vi "ScanningWaveform_v6.vi"(0 "Vy-min":dbl, 1 "Vy-max":dbl, 2 "yPixels/tPixels":dbl, 3 "xPixels/rPixels":dbl, 4 "Vx-min":dbl, 5 "Vx-max":dbl, 6 "Drawing Mode":u16(ring) items=["Image", "Fill Rectangle", "Fill Circle", "Draw Freeform", "Fill Freeform", "Ellipse Boundary", "Line"], 7 "Angle":dbl, 8 "Scanning Mode":u16(ring) items=["Raster", "Spiral"], 9 "AOrate":dbl, 10 "Points":cluster{"X":dbl, "Y":dbl}[](array[cluster]), 11 "points in ellipse":dbl) -> (12 "numPixels":dbl, 13 "Y-WaveArray":dbl[](array[numeric]), 14 "P":dbl, 19 "X-WaveArray":dbl[](array[numeric]))   [LabVIEW 2015]
panel:
  out "Y Graph 4":dbl[][](graph)
  out "Y Graph 3":dbl[][](graph)
  out "X-Y Graph 3":T1(graph)
  out "Y Graph 2":dbl[](graph)
  out "X-Y Graph 2":cluster{dbl[], dbl[]}(graph)
  out "min":dbl
  out "max":dbl
  out "Points 2":cluster{"R":dbl, "Theta":dbl}[](array[cluster])
  out "X-Y Graph":cluster{dbl[], dbl[]}(graph)
  out "flyback time (us)":dbl
  out "Y Graph":dbl[](graph)
  out "X Graph":dbl[](graph)
  out "C":dbl
  out "Sx":dbl
  out "S":dbl
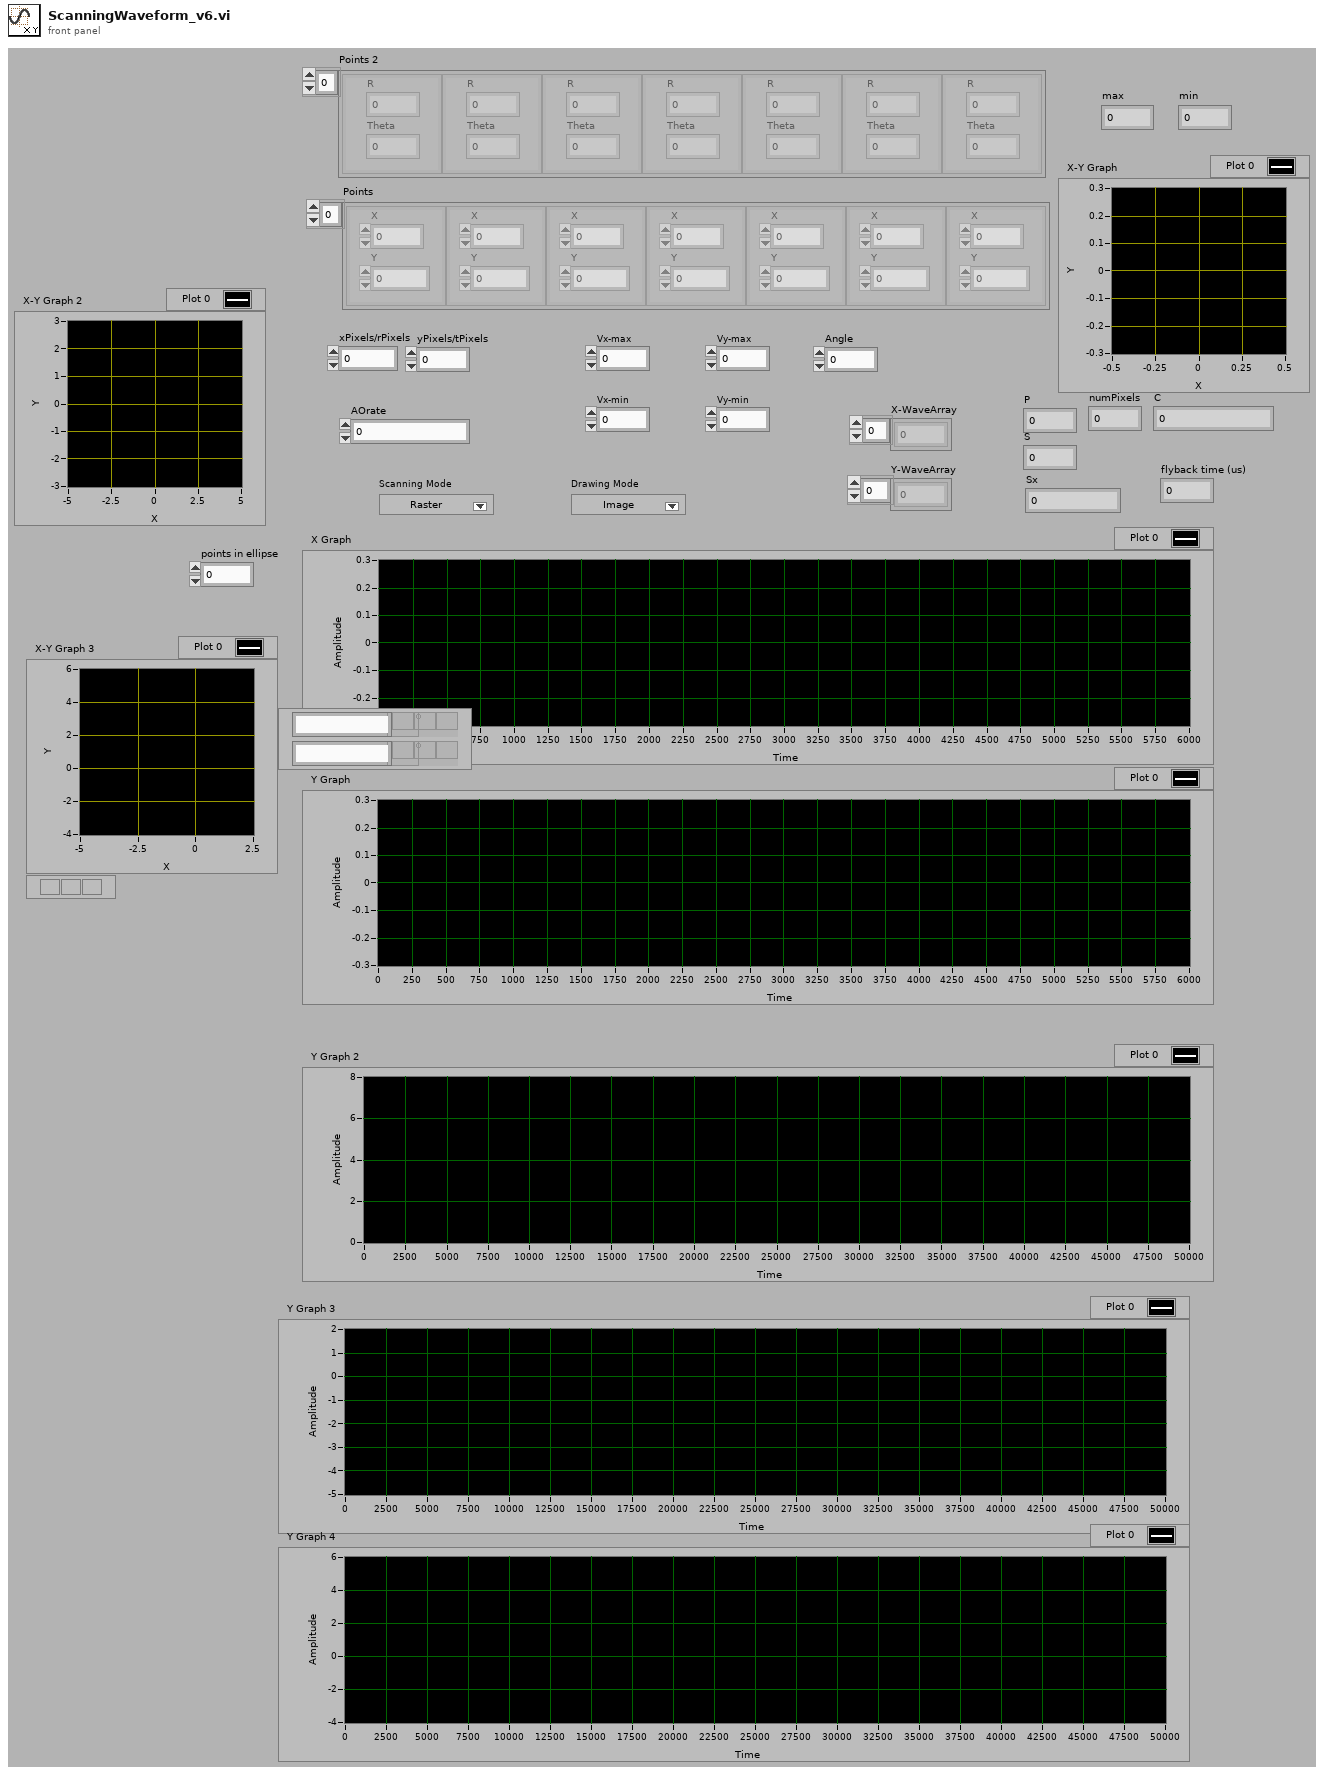
[diagram p1: front panel]
types:
  T1 = cluster{"X-WaveArray":dbl[], "Y-WaveArray":dbl[]}[]
  T2 = typedef "LVRectTypeDef.ctl" = cluster{"Left":i16, "Top":i16, "Right":i16, "Bottom":i16}
  T3 = cluster{"Xpixels":i32, "Vxminref":dbl, "Vxmaxref":dbl, "P":dbl, "Ypixels":i32, "Vyminref":dbl, "Vymaxref":dbl, "srate":sgl, "sAOxy":i32, "timeout":dbl, "type":string, "date":string, "time":string, "Colormap":u16, "Drawing Mode":u16, "Scanning Mode":u16, "square pixels":bool, "square matrix":bool, "Xpixels Img":i32, "Vx-min Img":dbl, "VX-max Img":dbl, "Ypixels Img":i32, "Vy-min Img":dbl, "Vy-max Img ":dbl, "Angle Img":dbl, "autoshutter":bool, "finite":bool, "cont":bool, "wavdet":bool, "measpoints":i32, "avpp":i32, "bufferAO":i32, "bufferAI":i32, "starttick":u32, "waveform":path, "Vx-ref":dbl, "Vy-ref":dbl, "refreshrate":dbl, "refreshbuffer":i32, "tt_cycles":i32, "motorref":refnum<k7>, "mirrorswitch":refnum<k7>, "sample mode":i32, "maxbufferAI":i32, "sampletreshold":dbl, "srateAODO":sgl, "bin":sgl, "Pel":sgl, "Angle draw":dbl, "srate Img":sgl, "ROIimg_plotbounds":T2, "auto OD":bool, "ODfilt":u16, "reset AO_DO":bool, "aAI":i32[], "aCI":i32[], "aAO":u32[], "aDO":u32[], "refwfsize":dbl, "Lifetime":bool, "Vz-Img":dbl, "Vz-ref":dbl, "Vz-reset":dbl}
  T4 = cluster{cluster{dbl, dbl}[], cluster{dbl, dbl}[]}
  T5 = cluster{"X-WaveArray":dbl[], "Y-WaveArray":dbl[]}
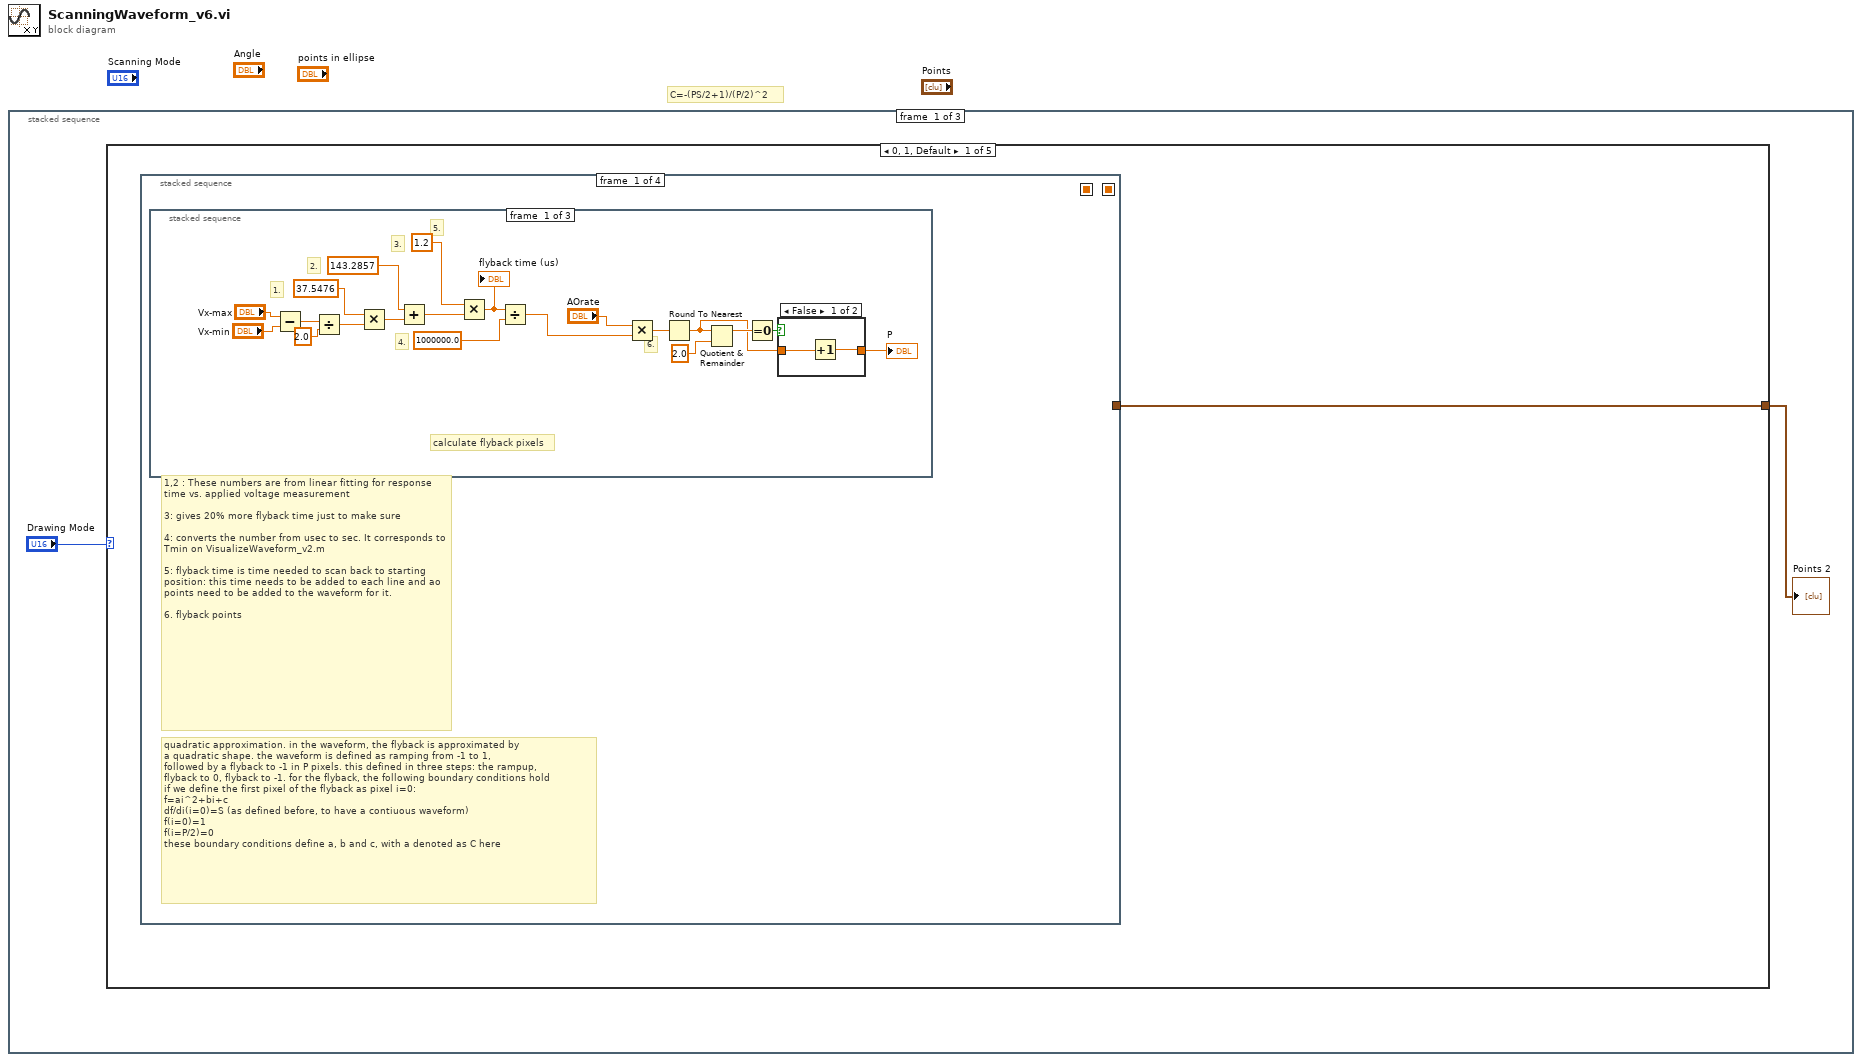
[diagram p0: block diagram]
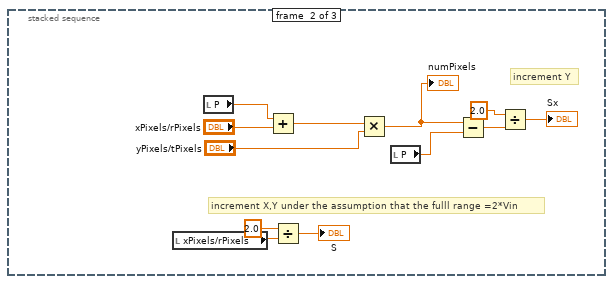
[diagram p3: hidden frame]
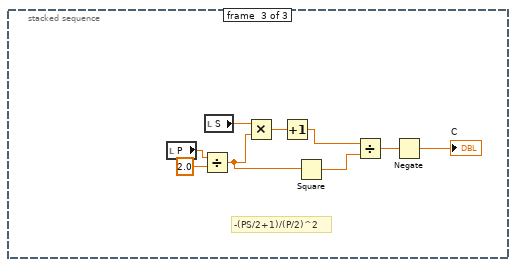
[diagram p4: hidden frame]
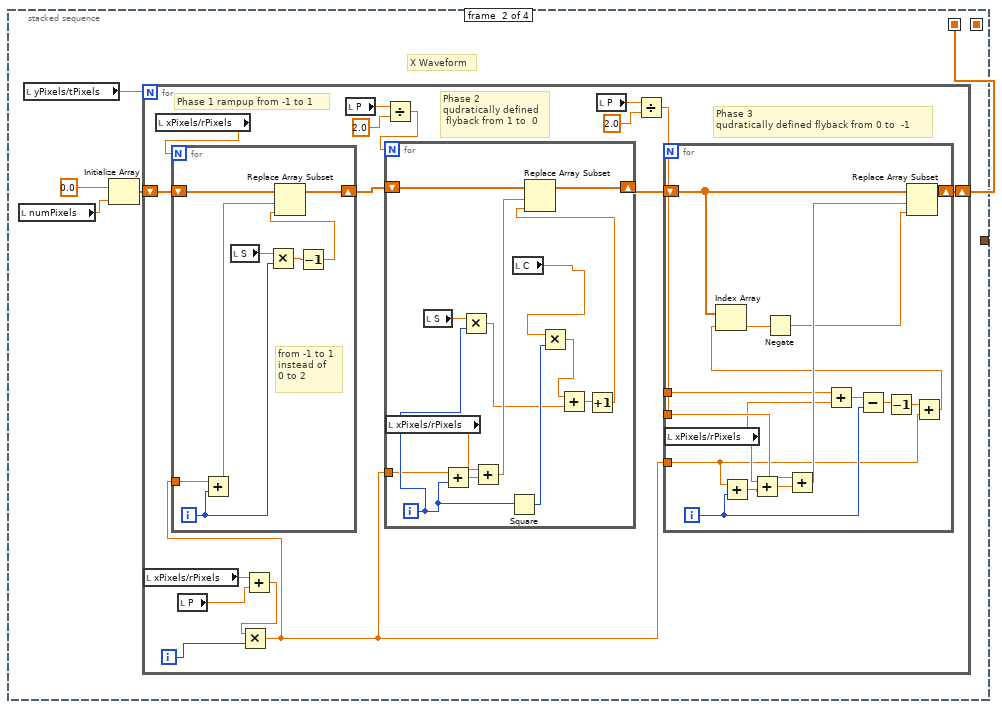
[diagram p5: hidden frame]
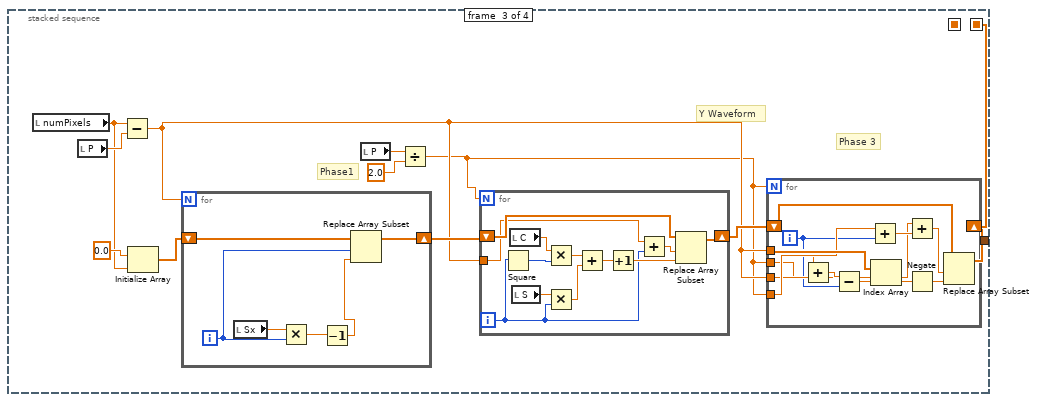
[diagram p6: hidden frame]
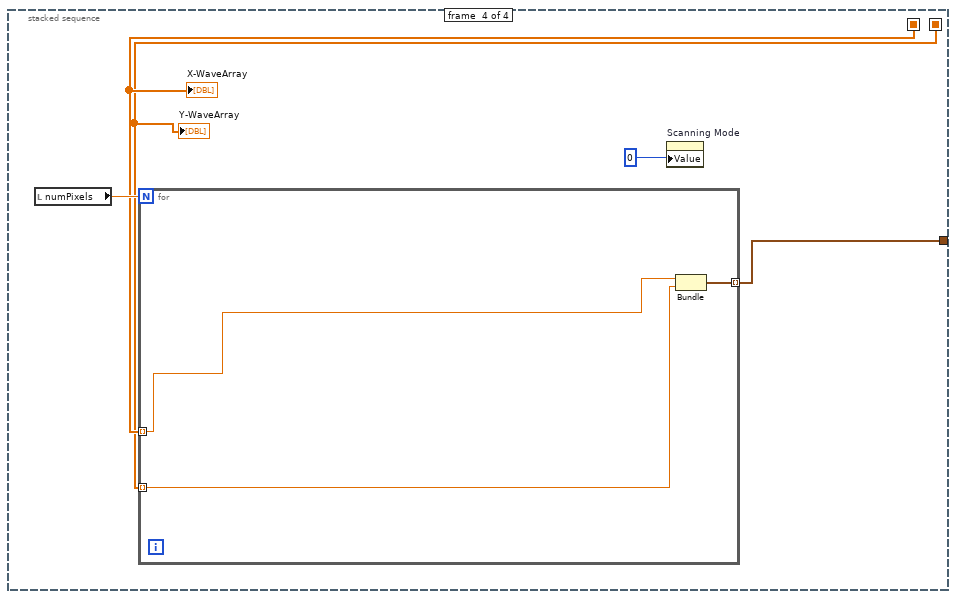
[diagram p7: hidden frame]
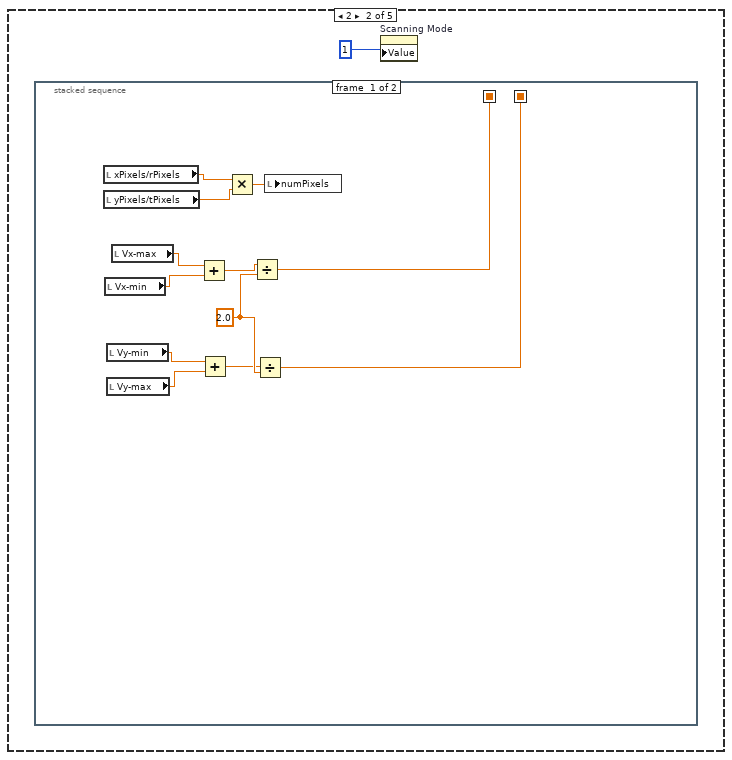
[diagram p8: hidden frame]
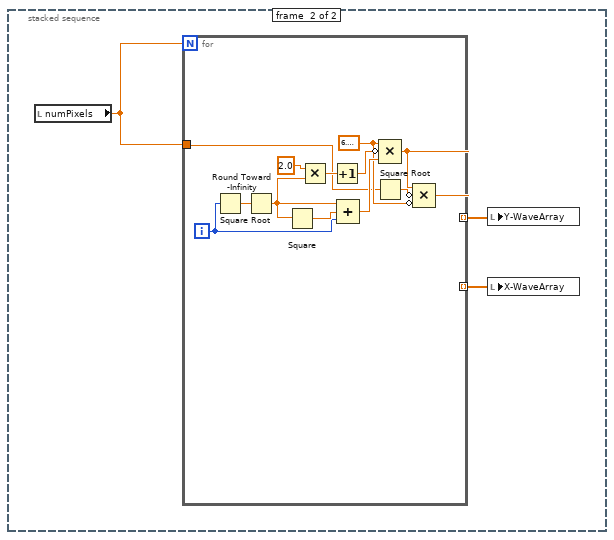
[diagram p9: hidden frame]
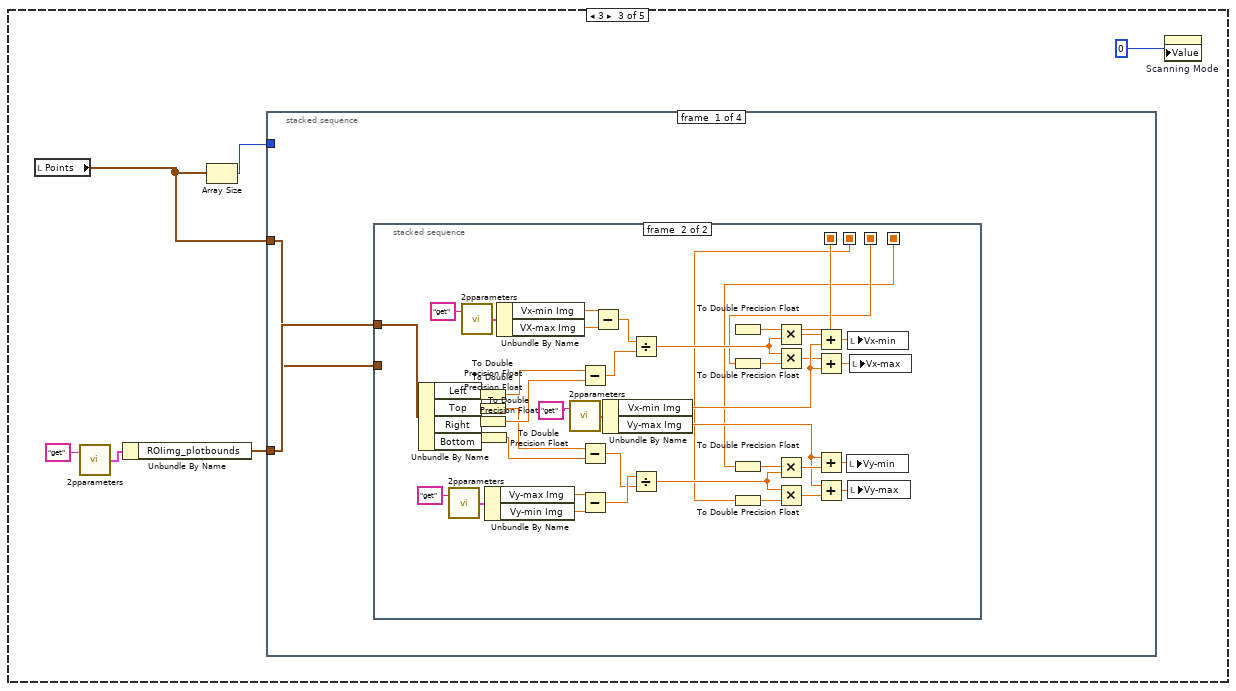
[diagram p10: hidden frame]
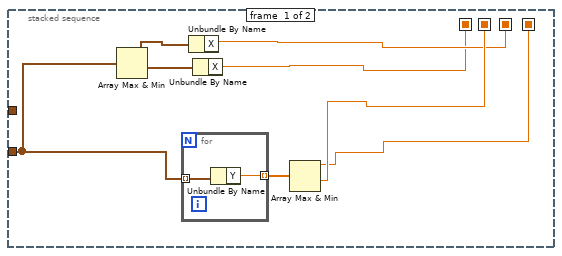
[diagram p11: hidden frame]
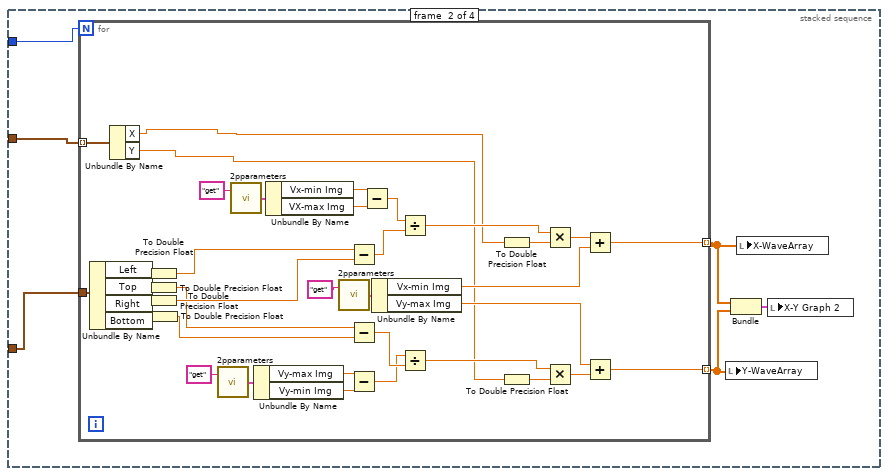
[diagram p12: hidden frame]
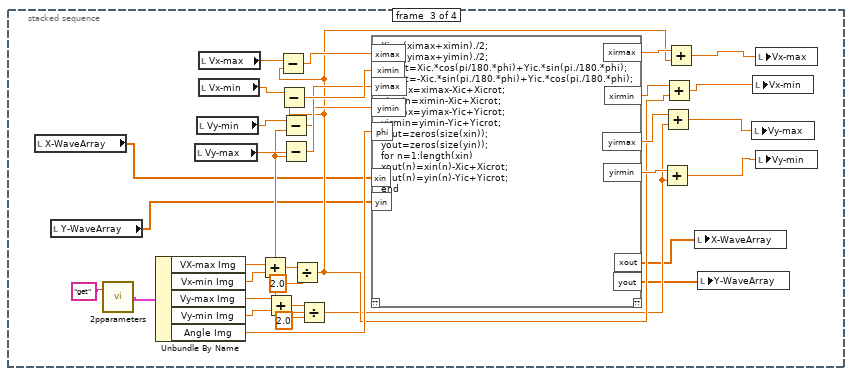
[diagram p13: hidden frame]
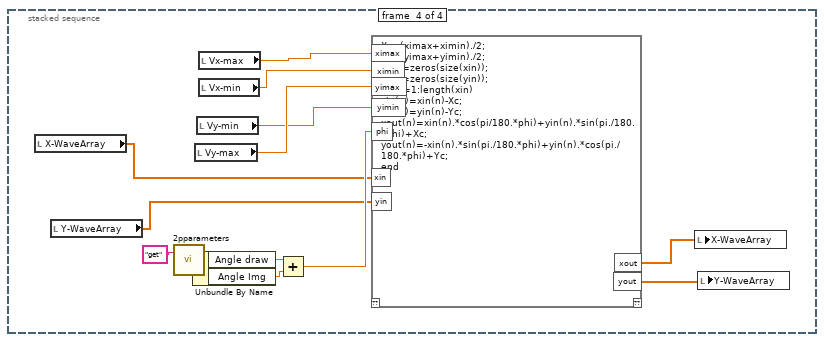
[diagram p14: hidden frame]
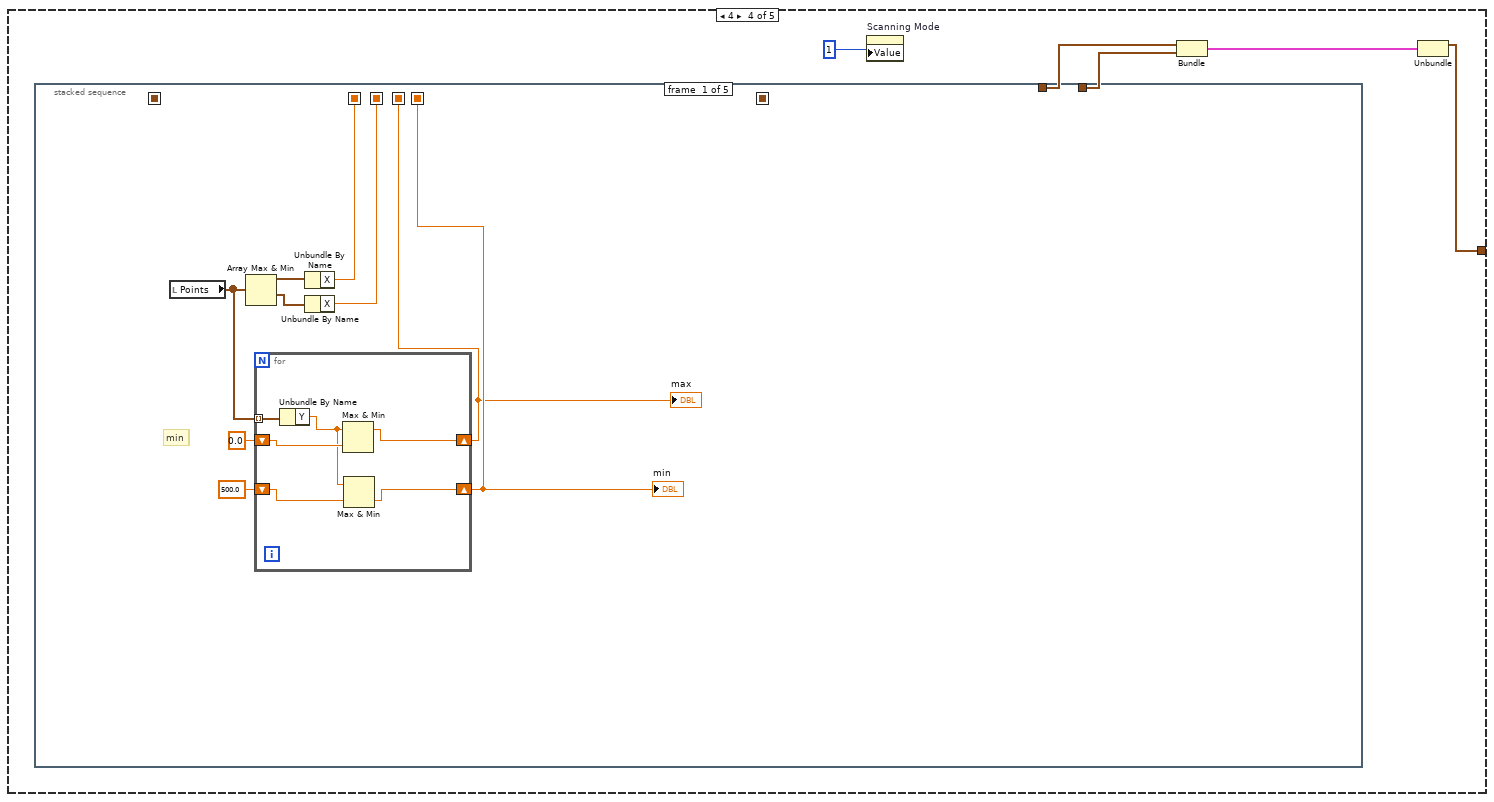
[diagram p15: hidden frame]
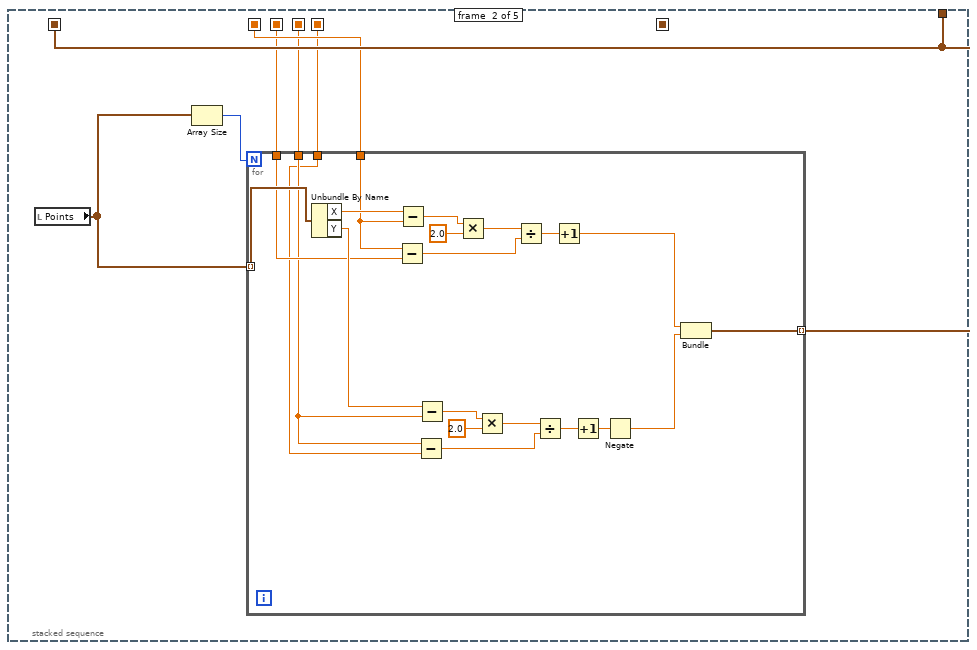
[diagram p16: hidden frame]
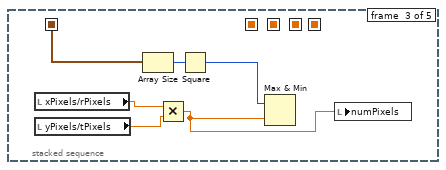
[diagram p17: hidden frame]
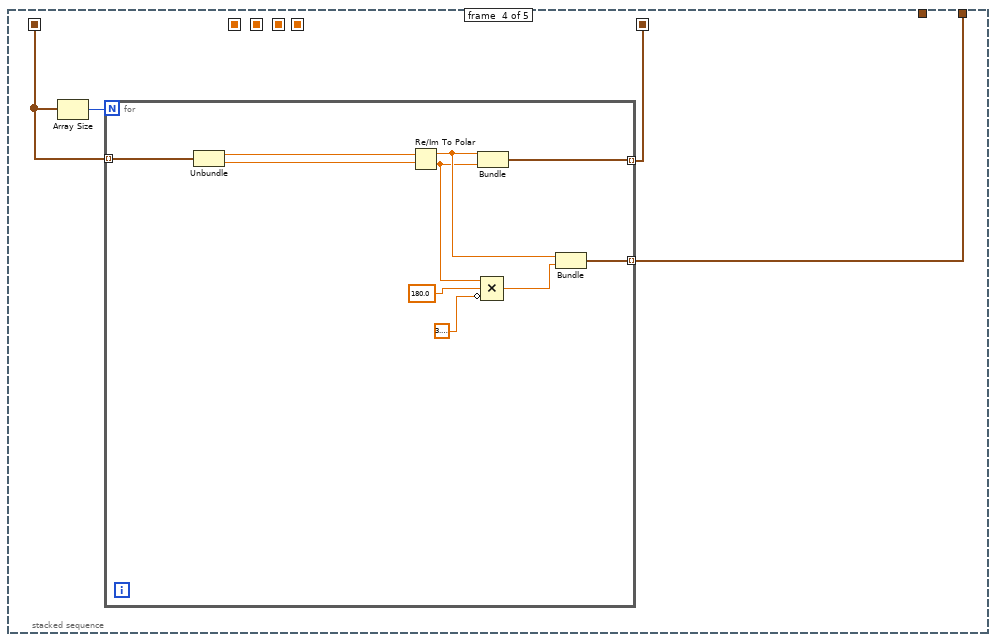
[diagram p18: hidden frame]
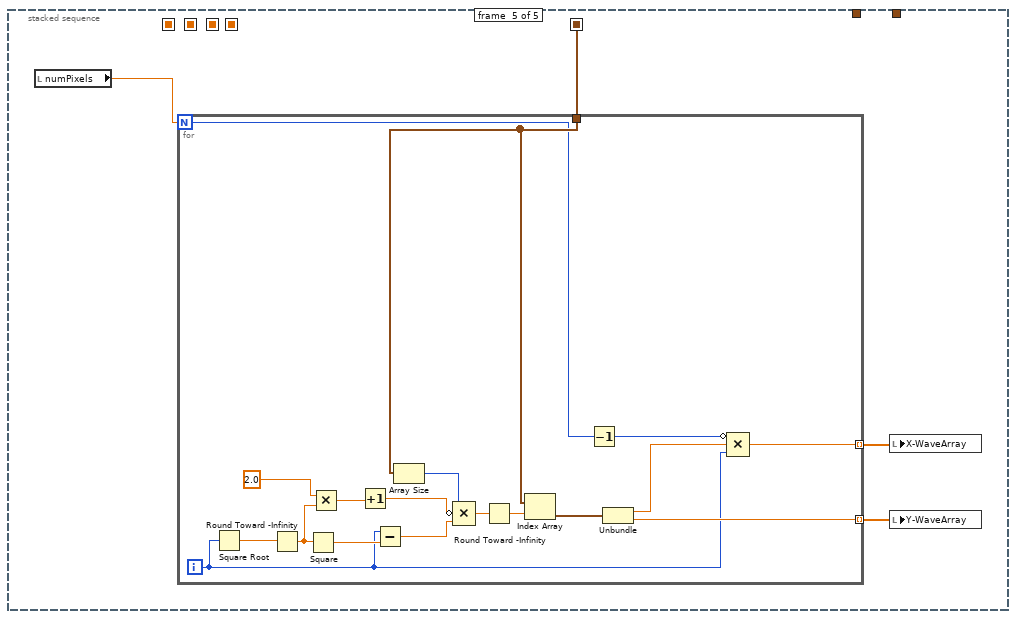
[diagram p19: hidden frame]
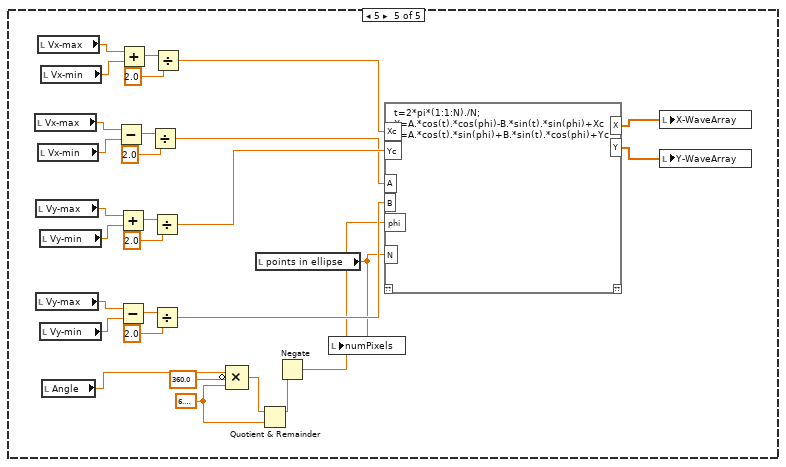
[diagram p20: hidden frame]
diagram:
  # "C=-(PS/2+1)/(P/2)^2"
  n1 = stacked-sequence {
    frame #0 {
      n2 = case shown="0, 1, Default" "Drawing Mode" {
        tunnel: [w3 _ _ w336 _] -> w1
        frame 0, 1, Default {
          n3 = stacked-sequence {
            seq-local: [_ w48 _ _] -> [_ _ _ w150]
            seq-local: [_ _ w107 _] -> [_ _ _ w149]
            tunnel: [_ _ _ w151] -> w3
            frame #0 {
              # "quadratic approximation. in the waveform, the flyback is approximated by\na quadratic shape. the waveform is defined as ramping from -1 to 1, \nfollowed by a flyback to -1 in P pixels. this defined in three steps: the rampup,\nflyback to 0, flyback to -1. for the flyback, the following boundary conditions hold\nif we define the first pixel of the flyback as pixel i=0:\nf=ai^2+bi+c\ndf/di(i=0)=S (as defined before, to have a contiuous waveform)\nf(i=0)=1\nf(i=P/2)=0\nthese boundary conditions define a, b and c, with a denoted as C here"
              # "1,2 : These numbers are from linear fitting for response time vs. applied voltage measurement\n\n3: gives 20% more flyback time just to make sure\n\n4: converts the number from usec to sec. It corresponds to Tmin on VisualizeWaveform_v2.m\n\n5: flyback time is time needed to scan back to starting position: this time needs to be added to each line and ao points need to be added to the waveform for it.\n\n6. flyback points"
              n4 = stacked-sequence {
                frame #0 {
                  # "calculate flyback pixels"
                  # "6."
                  # "5."
                  # "4."
                  # "3."
                  # "2."
                  # "1."
                  n5 = Subtract(x="Vx-max", y="Vx-min") -> (x-y=w5:dbl)
                  n6 = Divide(x=w5, y=2.0 ("x-y")) -> (x/y=w4:dbl)
                  n7 = Multiply(x=37.5476, y=w4) -> (x*y=w21:dbl)
                  n8 = Add(x=143.2857, y=w21) -> (x+y=w19:dbl)
                  n9 = Multiply(x=1.2, y=w19) -> (x*y=w17:dbl)
                  "flyback time (us)" <- w17
                  n10 = Divide(x=w17, y=1000000.0 ("x")) -> (x/y=w15:dbl)
                  n11 = Multiply(x="AOrate", y=w15) -> (x*y=w14:dbl)
                  n12 = Round To Nearest(number=w14) -> (nearest integer value=w9:dbl)
                  n13 = Quotient & Remainder(x=w9, y=2.0) -> (x-y*floor(x/y)=w11:dbl)  [unwired: 1 out]
                  n14 = Equal To 0?(x=w11) -> (x = 0?=w12:bool)
                  n15 = case shown="False" w12 {
                    tunnel: [w24 w26] -> w10
                    tunnel: w9 -> [w25 w26]
                    frame False {
                      n16 = Increment(x=w25) -> (x+1=w24:dbl)
                    }
                    frame True {
                    }
                  }
                  "P" <- w10
                }
                frame #1 {
                  # "increment X,Y under the assumption that the fulll range =2*Vin"
                  # "increment Y"
                  n17 = local read "xPixels/rPixels"() -> (w31:dbl)
                  n18 = local read "P"() -> (w37:dbl)
                  n19 = Add(x=w37, y="xPixels/rPixels") -> (x+y=w33:dbl)
                  n20 = Divide(x=2.0, y=w31) -> (x/y=→"S":dbl)
                  n21 = Multiply(x=w33, y="yPixels/tPixels") -> (x*y=w36:dbl)
                  "numPixels" <- w36
                  n22 = local read "P"() -> (w38:dbl)
                  n23 = Subtract(x=w36, y=w38) -> (x-y=w29:dbl)
                  n24 = Divide(x=2.0, y=w29) -> (x/y=→"Sx":dbl)
                }
                frame #2 {
                  # "-(PS/2+1)/(P/2)^2"
                  n25 = local read "P"() -> (w45:dbl)
                  n26 = Divide(x=w45, y=2.0) -> (x/y=w47:dbl)
                  n27 = local read "S"() -> (w46:dbl)
                  n28 = Multiply(x=w46, y=w47) -> (x*y=w42:dbl)
                  n29 = Increment(x=w42) -> (x+1=w39:dbl)
                  n30 = Square(x=w47) -> (x^2=w43:dbl)
                  n31 = Divide(x=w39, y=w43) -> (x/y=w44:dbl)
                  n32 = Negate(x=w44) -> (-x=→"C":dbl)
                }
              }
            }
            frame #1 {
              # "X Waveform"
              n33 = local read "numPixels"() -> (w50:dbl)
              n34 = local read "yPixels/tPixels"() -> (w52:dbl)
              n35 = Initialize Array(0.0 ("element"), w50) -> (w49:dbl[])
              n36 = for {
                N: w52 -> [_]
                shift-right: [w54] -> w48
                shift-left: w49 -> [w63]
                i -> [w68]
                # "Phase 3\nqudratically defined flyback from 0 to  -1"
                # "Phase 2\nqudratically defined\n flyback from 1 to  0"
                # "Phase 1 rampup from -1 to 1"
                n37 = local read "xPixels/rPixels"() -> (w67:dbl)
                n38 = local read "xPixels/rPixels"() -> (w64:dbl)
                n39 = local read "P"() -> (w66:dbl)
                n40 = Add(x=w67, y=w66) -> (x+y=w65:dbl)
                n41 = Multiply(x=w65, y=w68) -> (x*y=w53:dbl)
                n42 = for {
                  N: w64 -> [_]
                  shift-right: [w102] -> w55
                  shift-left: w63 -> [w106]
                  tunnel: w53 -> [w101]
                  i -> [w103]
                  # "from -1 to 1\ninstead of\n0 to 2"
                  n43 = Add(x=w101, y=w103) -> (x+y=w105:dbl)
                  n44 = local read "S"() -> (w104:dbl)
                  n45 = Multiply(x=w104, y=w103) -> (x*y=w100:dbl)
                  n46 = Decrement(x=w100) -> (x-1=w99:dbl)
                  n47 = Replace Array Subset(array=w106, new element=w99, index=w105) -> (w102:dbl[])
                }
                n48 = local read "P"() -> (w61:dbl)
                n49 = Divide(x=w61, y=2.0) -> (x/y=w62:dbl)
                n50 = for {
                  N: w62 -> [_]
                  shift-right: [w87] -> w57
                  shift-left: w55 -> [w98]
                  tunnel: w53 -> [w86]
                  i -> [w91]
                  n51 = local read "xPixels/rPixels"() -> (w96:dbl)
                  n52 = local read "S"() -> (w92:dbl)
                  n53 = Add(x=w86, y=w91) -> (x+y=w97:dbl)
                  n54 = Multiply(x=w92, y=w91) -> (x*y=w90:dbl)
                  n55 = Add(x=w96, y=w97) -> (x+y=w95:dbl)
                  n56 = Square(x=w91) -> (x^2=w94:i32)
                  n57 = local read "C"() -> (w85:dbl)
                  n58 = Multiply(x=w85, y=w94) -> (x*y=w93:dbl)
                  n59 = Add(x=w93, y=w90) -> (x+y=w89:dbl)
                  n60 = Increment(x=w89) -> (x+1=w88:dbl)
                  n61 = Replace Array Subset(array=w98, new element=w88, index=w95) -> (w87:dbl[])
                }
                n62 = local read "P"() -> (w58:dbl)
                n63 = Divide(x=w58, y=2.0) -> (x/y=w56:dbl)
                n64 = for {
                  N: w56 -> [_]
                  tunnel: w56 -> [w82]
                  tunnel: w56 -> [w79]
                  shift-right: [w70] -> w54
                  shift-left: w57 -> [w80]
                  tunnel: w53 -> [w69]
                  i -> [w76]
                  n65 = local read "xPixels/rPixels"() -> (w78:dbl)
                  n66 = Add(x=w69, y=w76) -> (x+y=w84:dbl)
                  n67 = Add(x=w78, y=w84) -> (x+y=w83:dbl)
                  n68 = Add(x=w82, y=w83) -> (x+y=w81:dbl)
                  n69 = Add(x=w79, y=w78) -> (x+y=w77:dbl)
                  n70 = Subtract(x=w77, y=w76) -> (x-y=w75:dbl)
                  n71 = Decrement(x=w75) -> (x-1=w74:dbl)
                  n72 = Add(x=w74, y=w69) -> (x+y=w73:dbl)
                  n73 = Index Array(array=w80, index=w73) -> (element=w72:dbl)
                  n74 = Negate(x=w72) -> (-x=w71:dbl)
                  n75 = Replace Array Subset(array=w80, new element=w71, index=w81) -> (w70:dbl[])
                }
              }
            }
            frame #2 {
              # "Phase 3"
              # "Phase1"
              # "Y Waveform"
              n76 = local read "numPixels"() -> (w114:dbl)
              n77 = local read "P"() -> (w115:dbl)
              n78 = Subtract(x=w114, y=w115) -> (x-y=w109:dbl)
              n79 = Initialize Array(0.0 ("element"), w114) -> (w116:dbl[])
              n80 = for {
                N: w109 -> [_]
                shift-right: [w145] -> w111
                shift-left: w116 -> [w148]
                i -> [w146]
                n81 = local read "Sx"() -> (w147:dbl)
                n82 = Multiply(x=w147, y=w146) -> (x*y=w143:dbl)
                n83 = Decrement(x=w143) -> (x-1=w144:dbl)
                n84 = Replace Array Subset(array=w148, new element=w144, index=w146) -> (w145:dbl[])
              }
              n85 = local read "P"() -> (w113:dbl)
              n86 = Divide(x=w113, y=2.0) -> (x/y=w108:dbl)
              n87 = for {
                N: w108 -> [_]
                shift-right: [w135] -> w110
                shift-left: w111 -> [w142]
                tunnel: w109 -> [w134]
                i -> [w132]
                n88 = Square(x=w132) -> (x^2=w140:i32)
                n89 = local read "C"() -> (w131:dbl)
                n90 = local read "S"() -> (w133:dbl)
                n91 = Multiply(x=w131, y=w140) -> (x*y=w139:dbl)
                n92 = Multiply(x=w133, y=w132) -> (x*y=w138:dbl)
                n93 = Add(x=w139, y=w138) -> (x+y=w137:dbl)
                n94 = Increment(x=w137) -> (x+1=w136:dbl)
                n95 = Add(x=w134, y=w132) -> (x+y=w141:dbl)
                n96 = Replace Array Subset(array=w142, new element=w136, index=w141) -> (w135:dbl[])
              }
              n97 = for {
                N: w108 -> [_]
                shift-right: [w124] -> w107
                shift-left: w110 -> [w128]
                tunnel: w108 -> [w123]
                tunnel: w109 -> [w122]
                tunnel: w109 -> [w121]
                tunnel: w108 -> [w120]
                i -> [w118]
                n98 = Add(x=w121, y=w120) -> (x+y=w127:dbl)
                n99 = Subtract(x=w127, y=w118) -> (x-y=w119:dbl)
                n100 = Add(x=w123, y=w118) -> (x+y=w130:dbl)
                n101 = Index Array(array=w128, index=w119) -> (element=w126:dbl)
                n102 = Add(x=w122, y=w130) -> (x+y=w129:dbl)
                n103 = Negate(x=w126) -> (-x=w125:dbl)
                n104 = Replace Array Subset(array=w128, new element=w125, index=w129) -> (w124:dbl[])
              }
            }
            frame #3 {
              n105 = local read "numPixels"() -> (w153:dbl)
              n106 = for {
                N: w153 -> [_]
                tunnel: w150 -> [w155] mode=indexing
                tunnel: w149 -> [w154] mode=indexing
                tunnel: [w156] -> w151 mode=indexing
                n107 = Bundle("element"=w155, "element"=w154) -> (w156:cluster{"element":dbl, "element":dbl})  [unwired: 1 in]
              }
              n108 = property on="Scanning Mode" class="Ring (strict)"("Value"=0) -> ()  [unwired: 2 in, 2 out]
              "X-WaveArray" <- w150
              "Y-WaveArray" <- w149
            }
          }
        }
        frame 2 {
          n109 = stacked-sequence {
            seq-local: [w159 _] -> [_ _]
            seq-local: [w163 _] -> [_ _]
            frame #0 {
              w167 = 2.0
              n110 = local read "xPixels/rPixels"() -> (w169:dbl)
              n111 = local read "yPixels/tPixels"() -> (w168:dbl)
              n112 = local read "Vx-min"() -> (w165:dbl)
              n113 = local read "Vy-min"() -> (w162:dbl)
              n114 = local read "Vy-max"() -> (w161:dbl)
              n115 = local read "Vx-max"() -> (w166:dbl)
              n116 = Add(x=w166, y=w165) -> (x+y=w164:dbl)
              n117 = Add(x=w162, y=w161) -> (x+y=w160:dbl)
              n118 = Multiply(x=w169, y=w168) -> (x*y=w158:dbl)
              n119 = Divide(x=w164, y=w167) -> (x/y=w163:dbl)
              n120 = Divide(x=w160, y=w167) -> (x/y=w159:dbl)
              n121 = local write "numPixels"(w158) -> ()
            }
            frame #1 {
              n122 = local read "numPixels"() -> (w170:dbl)
              n123 = for {
                N: w170 -> [_]
                tunnel: w170 -> [w174]
                tunnel: [w179] -> w171 mode=indexing
                tunnel: [w180] -> w172 mode=indexing
                i -> [w177]
                w175 = 6.283185307179586
                n124 = Square Root(x=w177) -> (sqrt(x)=w185:dbl)
                n125 = Round Toward -Infinity(1:w185) -> (0:w176:dbl)
                n126 = Square(x=w176) -> (x^2=w184:dbl)
                n127 = Multiply(x=2.0, y=w176) -> (x*y=w183:dbl)
                n128 = Increment(x=w183) -> (x+1=w182:dbl)
                n129 = Compound Arithmetic op=ADD(w176, w184, w177) -> (w178:dbl)
                n130 = Square Root(x=w174) -> (sqrt(x)=w173:dbl)
                n131 = Compound Arithmetic op=MULTIPLY(w175, invert w182, w178) -> (w180:dbl)
                n132 = Compound Arithmetic op=MULTIPLY(w180, invert w173, invert w175) -> (w179:dbl)
              }
              n133 = local write "Y-WaveArray"(w172) -> ()
              n134 = local write "X-WaveArray"(w171) -> ()
            }
          }
          n135 = property on="Scanning Mode" class="Ring (strict)"("Value"=1) -> ()  [unwired: 2 in, 2 out]
        }
        frame 3 {
          n136 = local read "Points"() -> (w188:cluster{"X":dbl, "Y":dbl}[])
          n137 = call "2pparameters.vi"("command"="get") -> ("params out"=w186:T3)  [unwired: 1 in]
          n138 = Unbundle By Name(w186) -> ("ROIimg_plotbounds"=w187:T2)
          n139 = Array Size(array=w188) -> (size(s)=w189:i32)
          n140 = stacked-sequence {
            tunnel: w188 -> [w192 w251 _ _]
            tunnel: w187 -> [w193 w252 _ _]
            tunnel: w189 -> [_ w250 _ _]
            frame #0 {
              n141 = stacked-sequence {
                seq-local: [w194 _] -> [_ w208]
                seq-local: [w197 _] -> [_ w207]
                seq-local: [w195 _] -> [_ w206]
                seq-local: [w196 _] -> [_ w205]
                tunnel: w192 -> [w201 _]
                tunnel: w193 -> [_ w204]
                frame #0 {
                  n142 = Array Max & Min(array=w201) -> (max value=w200:cluster{"X":dbl, "Y":dbl}, min value=w199:cluster{"X":dbl, "Y":dbl})  [unwired: 2 out]
                  n143 = for {
                    tunnel: w201 -> [w203] mode=indexing
                    tunnel: [w202] -> w198 mode=indexing
                    n144 = Unbundle By Name(w203) -> ("Y"=w202:dbl)
                  }
                  n145 = Unbundle By Name(w200) -> ("X"=w195:dbl)
                  n146 = Unbundle By Name(w199) -> ("X"=w194:dbl)
                  n147 = Array Max & Min(array=w198) -> (max value=w196:dbl, min value=w197:dbl)  [unwired: 2 out]
                }
                frame #1 {
                  n148 = Unbundle By Name(w204) -> ("Left"=w209:i16, "Top"=w210:i16, "Right"=w211:i16, "Bottom"=w212:i16)
                  n149 = call "2pparameters.vi"("command"="get") -> ("params out"=w230:T3)  [unwired: 1 in]
                  n150 = call "2pparameters.vi"("command"="get") -> ("params out"=w218:T3)  [unwired: 1 in]
                  n151 = To Double Precision Float(number=w209) -> (double precision float=w245:dbl)
                  n152 = To Double Precision Float(number=w210) -> (double precision float=w213:dbl)
                  n153 = To Double Precision Float(number=w211) -> (double precision float=w246:dbl)
                  n154 = To Double Precision Float(number=w212) -> (double precision float=w214:dbl)
                  n155 = Unbundle By Name(w230) -> ("Vy-max Img"=w232:dbl, "Vy-min Img"=w233:dbl)
                  n156 = Unbundle By Name(w218) -> ("Vx-min Img"=w224:dbl, "VX-max Img"=w219:dbl)
                  n157 = call "2pparameters.vi"("command"="get") -> ("params out"=w223:T3)  [unwired: 1 in]
                  n158 = Subtract(x=w245, y=w246) -> (x-y=w215:dbl)
                  n159 = Subtract(x=w213, y=w214) -> (x-y=w216:dbl)
                  n160 = Subtract(x=w232, y=w233) -> (x-y=w234:dbl)
                  n161 = Subtract(x=w224, y=w219) -> (x-y=w220:dbl)
                  n162 = Unbundle By Name(w223) -> ("Vx-min Img"=w228:dbl, "Vy-max Img"=w236:dbl)
                  n163 = Divide(x=w220, y=w215) -> (x/y=w242:dbl)
                  n164 = Divide(x=w234, y=w216) -> (x/y=w243:dbl)
                  n165 = To Double Precision Float(number=w208) -> (double precision float=w241:dbl)
                  n166 = To Double Precision Float(number=w206) -> (double precision float=w226:dbl)
                  n167 = To Double Precision Float(number=w205) -> (double precision float=w235:dbl)
                  n168 = To Double Precision Float(number=w207) -> (double precision float=w244:dbl)
                  n169 = Multiply(x=w241, y=w242) -> (x*y=w225:dbl)
                  n170 = Multiply(x=w242, y=w226) -> (x*y=w227:dbl)
                  n171 = Multiply(x=w235, y=w243) -> (x*y=w237:dbl)
                  n172 = Multiply(x=w243, y=w244) -> (x*y=w238:dbl)
                  n173 = Add(x=w225, y=w228) -> (x+y=w221:dbl)
                  n174 = Add(x=w227, y=w228) -> (x+y=w229:dbl)
                  n175 = Add(x=w236, y=w237) -> (x+y=w239:dbl)
                  n176 = Add(x=w236, y=w238) -> (x+y=w240:dbl)
                  n177 = local write "Vy-min"(w239) -> ()
                  n178 = local write "Vx-min"(w221) -> ()
                  n179 = local write "Vy-max"(w240) -> ()
                  n180 = local write "Vx-max"(w229) -> ()
                }
              }
            }
            frame #1 {
              n181 = for {
                N: w250 -> [_]
                tunnel: w252 -> [w260]
                tunnel: w251 -> [w259] mode=indexing
                tunnel: [w256] -> w248 mode=indexing
                tunnel: [w255] -> w247 mode=indexing
                n182 = Unbundle By Name(w260) -> ("Left"=w288:i16, "Top"=w287:i16, "Right"=w286:i16, "Bottom"=w285:i16)
                n183 = Unbundle By Name(w259) -> ("X"=w254:dbl, "Y"=w253:dbl)
                n184 = To Double Precision Float(number=w288) -> (double precision float=w258:dbl)
                n185 = To Double Precision Float(number=w287) -> (double precision float=w257:dbl)
                n186 = To Double Precision Float(number=w286) -> (double precision float=w261:dbl)
                n187 = To Double Precision Float(number=w285) -> (double precision float=w284:dbl)
                n188 = call "2pparameters.vi"("command"="get") -> ("params out"=w271:T3)  [unwired: 1 in]
                n189 = call "2pparameters.vi"("command"="get") -> ("params out"=w280:T3)  [unwired: 1 in]
                n190 = Unbundle By Name(w271) -> ("Vy-max Img"=w269:dbl, "Vy-min Img"=w268:dbl)
                n191 = Unbundle By Name(w280) -> ("Vx-min Img"=w275:dbl, "VX-max Img"=w279:dbl)
                n192 = call "2pparameters.vi"("command"="get") -> ("params out"=w276:T3)  [unwired: 1 in]
                n193 = Subtract(x=w258, y=w261) -> (x-y=w283:dbl)
                n194 = Subtract(x=w257, y=w284) -> (x-y=w282:dbl)
                n195 = Subtract(x=w269, y=w268) -> (x-y=w267:dbl)
                n196 = Subtract(x=w275, y=w279) -> (x-y=w278:dbl)
                n197 = Unbundle By Name(w276) -> ("Vx-min Img"=w272:dbl, "Vy-max Img"=w266:dbl)
                n198 = Divide(x=w278, y=w283) -> (x/y=w264:dbl)
                n199 = Divide(x=w267, y=w282) -> (x/y=w263:dbl)
                n200 = To Double Precision Float(number=w254) -> (double precision float=w274:dbl)
                n201 = To Double Precision Float(number=w253) -> (double precision float=w262:dbl)
                n202 = Multiply(x=w264, y=w274) -> (x*y=w273:dbl)
                n203 = Multiply(x=w263, y=w262) -> (x*y=w265:dbl)
                n204 = Add(x=w273, y=w272) -> (x+y=w256:dbl)
                n205 = Add(x=w266, y=w265) -> (x+y=w255:dbl)
              }
              n206 = local write "Y-WaveArray"(w247) -> ()
              n207 = Bundle(w248, w247) -> (w249:cluster{dbl[], dbl[]})  [unwired: 1 in]
              n208 = local write "X-WaveArray"(w248) -> ()
              n209 = local write "X-Y Graph 2"(w249) -> ()
            }
            frame #2 {
              n210 = local read "X-WaveArray"() -> (w291:dbl[])
              n211 = local read "Y-WaveArray"() -> (w292:dbl[])
              n212 = call "2pparameters.vi"("command"="get") -> ("params out"=w304:T3)  [unwired: 1 in]
              n213 = Unbundle By Name(w304) -> ("VX-max Img"=w306:dbl, "Vx-min Img"=w307:dbl, "Vy-max Img"=w308:dbl, "Vy-min Img"=w309:dbl, "Angle Img"=w299:dbl)
              n214 = local read "Vy-max"() -> (w316:dbl)
              n215 = local read "Vy-min"() -> (w317:dbl)
              n216 = local read "Vx-max"() -> (w314:dbl)
              n217 = local read "Vx-min"() -> (w315:dbl)
              n218 = Add(x=w306, y=w307) -> (x+y=w310:dbl)
              n219 = Add(x=w308, y=w309) -> (x+y=w313:dbl)
              n220 = Divide(x=w310, y=2.0) -> (x/y=w294:dbl)
              n221 = Subtract(x=w314, y=w294) -> (x-y=w303:dbl)
              n222 = Subtract(x=w315, y=w294) -> (x-y=w302:dbl)
              n223 = Divide(x=w313, y=2.0) -> (x/y=w293:dbl)
              n224 = Subtract(x=w317, y=w293) -> (x-y=w300:dbl)
              n225 = Subtract(x=w316, y=w293) -> (x-y=w301:dbl)
              n226 = script code="Xic=(ximax+ximin)./2;\nYic=(yimax+yimin)./2;\nXicrot=Xic.*cos(pi/180.*phi)+Yic.*sin(pi./180.*phi);\nYicrot=-Xic.*sin(pi./180.*phi)+Yic.*cos(pi./180.*phi);\nxirmax=ximax-Xic+Xicrot;\nxirmin=ximin-Xic+Xicrot;\nyirmax=yimax-Yic+Yicrot;\nyirmin=yimin-Yic+Yicrot;\nxout=zeros(size(xin));\nyout=zeros(size(yin));\nfor n=1:length(xin)\nxout(n)=xin(n)-Xic+Xicrot;\nyout(n)=yin(n)-Yic+Yicrot;\nend"("ximax"=w303, "ximin"=w302, "yimax"=w301, "yimin"=w300, "phi"=w299, "xin"=w291, "yin"=w292) -> ("xirmax"=w298:dbl, "xirmin"=w297:dbl, "yirmax"=w296:dbl, "yirmin"=w295:dbl, "xout"=w290:dbl[], "yout"=w289:dbl[])  [unwired: 1 in, 1 out]
              n227 = Add(x=w295, y=w293) -> (x+y=w321:dbl)
              n228 = Add(x=w296, y=w293) -> (x+y=w320:dbl)
              n229 = Add(x=w297, y=w294) -> (x+y=w319:dbl)
              n230 = Add(x=w298, y=w294) -> (x+y=w318:dbl)
              n231 = local write "X-WaveArray"(w290) -> ()
              n232 = local write "Y-WaveArray"(w289) -> ()
              n233 = local write "Vy-max"(w320) -> ()
              n234 = local write "Vx-min"(w319) -> ()
              n235 = local write "Vx-max"(w318) -> ()
              n236 = local write "Vy-min"(w321) -> ()
            }
            frame #3 {
              n237 = local read "X-WaveArray"() -> (w324:dbl[])
              n238 = local read "Y-WaveArray"() -> (w325:dbl[])
              n239 = call "2pparameters.vi"("command"="get") -> ("params out"=w331:T3)  [unwired: 1 in]
              n240 = Unbundle By Name(w331) -> ("Angle draw"=w332:dbl, "Angle Img"=w333:dbl)
              n241 = local read "Vy-max"() -> (w329:dbl)
              n242 = local read "Vy-min"() -> (w328:dbl)
              n243 = local read "Vx-max"() -> (w326:dbl)
              n244 = local read "Vx-min"() -> (w327:dbl)
              n245 = Add(x=w332, y=w333) -> (x+y=w334:dbl)
              n246 = script code="Xc=(ximax+ximin)./2;\nYc=(yimax+yimin)./2;\nxout=zeros(size(xin));\nyout=zeros(size(yin));\nfor n=1:length(xin)\nxin(n)=xin(n)-Xc;\nyin(n)=yin(n)-Yc;\nxout(n)=xin(n).*cos(pi/180.*phi)+yin(n).*sin(pi./180.*phi)+Xc;\nyout(n)=-xin(n).*sin(pi./180.*phi)+yin(n).*cos(pi./180.*phi)+Yc;\nend"("ximax"=w326, "ximin"=w327, "yimax"=w329, "yimin"=w328, "phi"=w334, "xin"=w324, "yin"=w325) -> ("xout"=w323:dbl[], "yout"=w322:dbl[])  [unwired: 1 in, 1 out]
              n247 = local write "X-WaveArray"(w323) -> ()
              n248 = local write "Y-WaveArray"(w322) -> ()
            }
          }
          n249 = property on="Scanning Mode" class="Ring (strict)"("Value"=0) -> ()  [unwired: 2 in, 2 out]
        }
        frame 4 {
          n250 = stacked-sequence {
            seq-local: [_ _ _ w390 _] -> [_ _ _ _ w405]
            seq-local: [_ w359 _ _ _] -> [_ _ w384 w391 _]
            seq-local: [w345 _ _ _ _] -> [_ w358 _ _ _]
            seq-local: [w344 _ _ _ _] -> [_ w357 _ _ _]
            seq-local: [w342 _ _ _ _] -> [_ w356 _ _ _]
            seq-local: [w343 _ _ _ _] -> [_ w355 _ _ _]
            tunnel: [_ w359 _ _ _] -> w338
            tunnel: [_ _ _ w389 _] -> w337
            frame #0 {
              # "min"
              # "max"
              n251 = local read "Points"() -> (w346:cluster{"X":dbl, "Y":dbl}[])
              n252 = Array Max & Min(array=w346) -> (max value=w348:cluster{"X":dbl, "Y":dbl}, min value=w347:cluster{"X":dbl, "Y":dbl})  [unwired: 2 out]
              n253 = for {
                tunnel: w346 -> [w354] mode=indexing
                shift-right: [w350] -> w342
                shift-left: 0.0 -> [w353]
                shift-right: [w349] -> w343
                shift-left: 500.0 -> [w351]
                n254 = Unbundle By Name(w354) -> ("Y"=w352:dbl)
                n255 = Max & Min(x=w352, y=w353) -> (max(x,y)=w350:dbl)  [unwired: 1 out]
                n256 = Max & Min(x=w352, y=w351) -> (min(x,y)=w349:dbl)  [unwired: 1 out]
              }
              "max" <- w342
              "min" <- w343
              n257 = Unbundle By Name(w348) -> ("X"=w345:dbl)
              n258 = Unbundle By Name(w347) -> ("X"=w344:dbl)
            }
            frame #1 {
              n259 = local read "Points"() -> (w360:cluster{"X":dbl, "Y":dbl}[])
              n260 = Array Size(array=w360) -> (size(s)=w361:i32)
              n261 = for {
                N: w361 -> [_]
                tunnel: w360 -> [w382] mode=indexing
                tunnel: [w381] -> w359 mode=indexing
                tunnel: w358 -> [w367]
                tunnel: w357 -> [w366]
                tunnel: w356 -> [w365]
                tunnel: w355 -> [w364]
                n262 = Unbundle By Name(w382) -> ("X"=w369:dbl, "Y"=w368:dbl)
                n263 = Subtract(x=w367, y=w366) -> (x-y=w376:dbl)
                n264 = Subtract(x=w369, y=w367) -> (x-y=w377:dbl)
                n265 = Subtract(x=w365, y=w364) -> (x-y=w371:dbl)
                n266 = Subtract(x=w368, y=w365) -> (x-y=w372:dbl)
                n267 = Multiply(x=w377, y=2.0) -> (x*y=w378:dbl)
                n268 = Multiply(x=w372, y=2.0) -> (x*y=w373:dbl)
                n269 = Divide(x=w378, y=w376) -> (x/y=w380:dbl)
                n270 = Divide(x=w373, y=w371) -> (x/y=w374:dbl)
                n271 = Increment(x=w380) -> (x+1=w379:dbl)
                n272 = Increment(x=w374) -> (x+1=w363:dbl)
                n273 = Negate(x=w363) -> (-x=w362:dbl)
                n274 = Bundle(w379, w362) -> (w381:cluster{dbl, dbl})  [unwired: 1 in]
              }
            }
            frame #2 {
              n275 = local read "xPixels/rPixels"() -> (w388:dbl)
              n276 = local read "yPixels/tPixels"() -> (w387:dbl)
              n277 = Array Size(array=w384) -> (size(s)=w385:i32)
              n278 = Multiply(x=w388, y=w387) -> (x*y=w383:dbl)
              n279 = Square(x=w385) -> (x^2=w386:i32)
              n280 = Max & Min(x=w386, y=w383) -> ()  [unwired: 2 out]
              n281 = local write "numPixels"(w383) -> ()
            }
            frame #3 {
              n282 = Array Size(array=w391) -> (size(s)=w392:i32)
              n283 = for {
                N: w392 -> [_]
                tunnel: w391 -> [w402] mode=indexing
                tunnel: [w399] -> w390 mode=indexing
                tunnel: [w398] -> w389 mode=indexing
                n284 = Unbundle(w402) -> (w401:dbl, w400:dbl)
                n285 = Re/Im To Polar(2:w400, 3:w401) -> (0:w393:dbl, 1:w397:dbl)
                n286 = Bundle(w397, w393) -> (w399:cluster{dbl, dbl})  [unwired: 1 in]
                n287 = Compound Arithmetic op=MULTIPLY(w393, 180.0, invert 3.141592653589793) -> (w396:dbl)
                n288 = Bundle(w397, w396) -> (w398:cluster{dbl, dbl})  [unwired: 1 in]
              }
            }
            frame #4 {
              n289 = local read "numPixels"() -> (w406:dbl)
              n290 = for {
                N: w406 -> [w408]
                tunnel: w405 -> [w415]
                tunnel: [w413] -> w404 mode=indexing
                tunnel: [w412] -> w403 mode=indexing
                i -> [w410]
                n291 = Square Root(x=w410) -> (sqrt(x)=w423:dbl)
                n292 = Round Toward -Infinity(1:w423) -> (0:w421:dbl)
                n293 = Square(x=w421) -> (x^2=w422:dbl)
                n294 = Multiply(x=2.0, y=w421) -> (x*y=w420:dbl)
                n295 = Increment(x=w420) -> (x+1=w418:dbl)
                n296 = Subtract(x=w410, y=w422) -> (x-y=w417:dbl)
                n297 = Array Size(array=w415) -> (size(s)=w419:i32)
                n298 = Compound Arithmetic op=MULTIPLY(w419, invert w418, w417) -> (w411:dbl)
                n299 = Round Toward -Infinity(1:w411) -> (0:w409:dbl)
                n300 = Index Array(array=w415, index=w409) -> (element=w424:cluster{dbl, dbl})
                n301 = Decrement(x=w408) -> (x-1=w407:i32)
                n302 = Unbundle(w424) -> (w416:dbl, w413:dbl)
                n303 = Compound Arithmetic op=MULTIPLY(invert w407, w416, w410) -> (w412:dbl)
              }
              n304 = local write "X-WaveArray"(w403) -> ()
              n305 = local write "Y-WaveArray"(w404) -> ()
            }
          }
          n306 = property on="Scanning Mode" class="Ring (strict)"("Value"=u16 1) -> ()  [unwired: 2 in, 2 out]
          n307 = Bundle(w338, w337) -> (w339:T4)  [unwired: 1 in]
          n308 = Unbundle(w339) -> (w336:cluster{dbl, dbl}[])  [unwired: 1 out]
        }
        frame 5 {
          w430 = 6.283185307179586
          n309 = local read "Vx-max"() -> (w442:dbl)
          n310 = local read "Vy-max"() -> (w446:dbl)
          n311 = local read "Vy-max"() -> (w441:dbl)
          n312 = local read "Vx-max"() -> (w453:dbl)
          n313 = local read "Vx-min"() -> (w443:dbl)
          n314 = local read "Vy-min"() -> (w447:dbl)
          n315 = local read "Vy-min"() -> (w440:dbl)
          n316 = local read "Vx-min"() -> (w452:dbl)
          n317 = local read "Angle"() -> (w428:dbl)
          n318 = Subtract(x=w442, y=w443) -> (x-y=w444:dbl)
          n319 = Add(x=w446, y=w447) -> (x+y=w448:dbl)
          n320 = Subtract(x=w441, y=w440) -> (x-y=w439:dbl)
          n321 = Add(x=w453, y=w452) -> (x+y=w451:dbl)
          n322 = Divide(x=w444, y=2.0) -> (x/y=w436:dbl)
          n323 = Divide(x=w448, y=2.0) -> (x/y=w437:dbl)
          n324 = Divide(x=w439, y=2.0) -> (x/y=w435:dbl)
          n325 = Divide(x=w451, y=2.0) -> (x/y=w425:dbl)
          n326 = Compound Arithmetic op=MULTIPLY(w428, invert 360.0, w430) -> (w431:dbl)
          n327 = local read "points in ellipse"() -> (w432:dbl)
          n328 = Quotient & Remainder(x=w431, y=w430) -> (x-y*floor(x/y)=w427:dbl)  [unwired: 1 out]
          n329 = Negate(x=w427) -> (-x=w426:dbl)
          n330 = local write "numPixels"(w432) -> ()
          n331 = script code="t=2*pi*(1:1:N)./N;\nX=A.*cos(t).*cos(phi)-B.*sin(t).*sin(phi)+Xc\nY=A.*cos(t).*sin(phi)+B.*sin(t).*cos(phi)+Yc"("Xc"=w425, "Yc"=w437, "A"=w436, "B"=w435, "phi"=w426, "N"=w432) -> ("X"=w434:dbl[], "Y"=w433:dbl[])  [unwired: 1 in, 1 out]
          n332 = local write "X-WaveArray"(w434) -> ()
          n333 = local write "Y-WaveArray"(w433) -> ()
        }
      }
      "Points 2" <- w1
    }
    frame #1 {
      n334 = local read "Drawing Mode"() -> (w454:u16)
      n335 = case shown="0, Default" w454 {
        frame 0, Default {
          n336 = flat-sequence {
            tunnel: [w460] -> w457
            tunnel: [w461] -> w458
            tunnel: [w486] -> w456
            tunnel: [w487] -> w455
            tunnel: w458 -> [w488]
            tunnel: w457 -> [w489]
            tunnel: w456 -> [w503]
            tunnel: w455 -> [w502]
            frame #0 {
              n337 = local read "Scanning Mode"() -> (w459:u16)
              n338 = case shown="0, Default" w459 {
                tunnel: [w464 w466] -> w460
                tunnel: [w463 w465] -> w461
                frame 0, Default {
                  # "-1<x<1\n-1<y<1"
                  n339 = local read "Y-WaveArray"() -> (w463:dbl[])
                  n340 = local read "X-WaveArray"() -> (w464:dbl[])
                  n341 = Bundle("X-WaveArray"=w464, "Y-WaveArray"=w463) -> (→"X-Y Graph 2":T5)  [unwired: 1 in]
                }
                frame 1 {
                  # "0<x<1\n0<y<2pi"
                  n342 = local read "X-WaveArray"() -> (w467:dbl[])
                  n343 = local read "Y-WaveArray"() -> (w468:dbl[])
                  n344 = Polar To Re/Im(2:w468, 3:w467) -> (0:w465:dbl[], 1:w466:dbl[])
                }
              }
            }
            frame #1 {
              w471 = 2.0
              n345 = local read "Vy-min"() -> (w482:dbl)
              n346 = Subtract(x="Vy-max", y=w482) -> (x-y=w484:dbl)
              n347 = Compound Arithmetic op=MULTIPLY(invert w471, w484, w488) -> (w480:dbl[])
              n348 = local read "Vx-max"() -> (w477:dbl)
              n349 = local read "Vx-min"() -> (w485:dbl)
              n350 = Subtract(x=w477, y=w485) -> (x-y=w483:dbl)
              n351 = Compound Arithmetic op=MULTIPLY(w483, w489, invert w471) -> (w481:dbl[])
              n352 = for {
                tunnel: [w497] -> w479 mode=indexing
                tunnel: [w496] -> w478 mode=indexing
                tunnel: w481 -> [w495] mode=indexing
                tunnel: w480 -> [w494] mode=indexing
                n353 = local read "Angle"() -> (w493:dbl)
                n354 = Compound Arithmetic op=MULTIPLY(6.283185307179586, w493, invert 360.0) -> (w490:dbl)
                n355 = formula code="px = xs*cos(t)+ys*sin(t);\npy = -xs*sin(t)+ys*cos(t);"("xs"=w495, "ys"=w494, "t"=w490) -> ("px"=w497:dbl, "py"=w496:dbl)
              }
              n356 = Add(x="Vy-min", y="Vy-max") -> (x+y=w472:dbl)
              n357 = local read "Vx-min"() -> (w476:dbl)
              n358 = Divide(x=w472, y=w471) -> (x/y=w473:dbl)
              n359 = Add(x=w477, y=w476) -> (x+y=w475:dbl)
              n360 = Add(x=w478, y=w473) -> (x+y=w487:dbl[])
              n361 = Divide(x=w475, y=w471) -> (x/y=w474:dbl)
              n362 = Add(x=w479, y=w474) -> (x+y=w486:dbl[])
            }
            frame #2 {
              n363 = local write "X-WaveArray"(w503) -> ()
              n364 = Bundle(w503, w502) -> (→"X-Y Graph":cluster{dbl[], dbl[]})  [unwired: 1 in]
              n365 = property on="X-Y Graph" class="XYGraph (strict)"("XScale.Maximum"=10.0 ("X Scale.Range:Maximum"), "XScale.Minimum"=-10.0 ("X Scale.Range:Minimum"), "YScale.Maximum"=10.0 ("Y Scale.Range:Maximum"), "YScale.Minimum"=-10.0 ("Y Scale.Range:Minimum")) -> ()  [unwired: 2 in, 2 out]
              n366 = local write "Y-WaveArray"(w502) -> ()
              "X Graph" <- w503
              "Y Graph" <- w502
            }
          }
        }
        frame 3, 5 {
          n367 = local read "Y-WaveArray"() -> (w505:dbl[])
          n368 = local read "X-WaveArray"() -> (w506:dbl[])
          n369 = Bundle("X-WaveArray"=w506, "Y-WaveArray"=w505) -> (w507:T5)  [unwired: 1 in]
          n370 = local write "Y Graph"(w505) -> ()
          n371 = local write "X-Y Graph"(w507) -> ()
          n372 = local write "X Graph"(w506) -> ()
        }
      }
    }
    frame #2 {
      n373 = local read "Drawing Mode"() -> (w508:u16)
      n374 = case shown="3" w508 {
        frame 0, Default {
        }
        frame 3 {
          n375 = local read "X-WaveArray"() -> (w525:dbl[])
          n376 = local read "Y-WaveArray"() -> (w524:dbl[])
          n377 = local read "points in ellipse"() -> (w509:dbl)
          n378 = Array Size(array=w525) -> (size(s)=w536:i32)
          n379 = local read "points in ellipse"() -> (w532:dbl)
          n380 = Array Size(array=w524) -> (size(s)=w528:i32)
          n381 = Decrement(x=w536) -> (x-1=w535:i32)
          n382 = Decrement(x=w528) -> (x-1=w529:i32)
          n383 = To Double Precision Float(number=w535) -> (double precision float=w534:dbl)
          n384 = local write "numPixels"(w509) -> ()
          n385 = To Double Precision Float(number=w529) -> (double precision float=w530:dbl)
          n386 = Divide(x=w534, y=w509) -> (x/y=w533:dbl)
          n387 = Divide(x=w530, y=w532) -> (x/y=w531:dbl)
          n388 = for {
            N: w509 -> [_]
            tunnel: w525 -> [w571]
            tunnel: w533 -> [w570]
            tunnel: [w569] -> w527 mode=indexing
            i -> [w567]
            n389 = Multiply(x=w570, y=w567) -> (x*y=w568:dbl)
            n390 = Interpolate 1D Array(1:w568, 2:w571) -> (0:w569:dbl)
          }
          n391 = for {
            N: w532 -> [_]
            tunnel: w524 -> [w566]
            tunnel: w531 -> [w565]
            tunnel: [w564] -> w526 mode=indexing
            i -> [w562]
            n392 = Multiply(x=w565, y=w562) -> (x*y=w563:dbl)
            n393 = Interpolate 1D Array(1:w563, 2:w566) -> (0:w564:dbl)
          }
          n394 = Bundle("X-WaveArray"=w525, "Y-WaveArray"=w524) -> (w542:T5)  [unwired: 1 in]
          n395 = Rotate 1D Array(1:w527, 2:1 ("n")) -> (0:w550:dbl[])
          n396 = Rotate 1D Array(1:w526, 2:1 ("n")) -> (0:w549:dbl[])
          n397 = Subtract(x=w527, y=w550) -> (x-y=w547:dbl[])
          n398 = Subtract(x=w526, y=w549) -> (x-y=w546:dbl[])
          n399 = Square(x=w547) -> (x^2=w545:dbl[])
          n400 = Square(x=w546) -> (x^2=w544:dbl[])
          n401 = Add(x=w545, y=w544) -> (x+y=w543:dbl[])
          n402 = Square Root(x=w543) -> (sqrt(x)=w539:dbl[])
          "Y Graph 2" <- w539
          n403 = script code="a=dr2<0.00;\nwhile sum(a)>0\nb=diff(a);\nx=x(b<1);\ny=y(b<1);\nx=[x(end) x];\ny=[y(end) y];\ndr2=sqrt((diff(x)).^2+(diff(y)).^ 2)\na=dr2<0.0;\nend\nxout=x;\nyout=y;"("dr2"=w539, "x"=w527, "y"=w526) -> ("xout"=w518:dbl[], "yout"=w510:dbl[])  [unwired: 1 in, 1 out]
          n404 = Bundle(w518, w510) -> (w541:cluster{dbl[], dbl[]})  [unwired: 1 in]
          n405 = Build Array(w527, w518) -> (→"Y Graph 3":dbl[][])
          n406 = Build Array(w526, w510) -> (→"Y Graph 4":dbl[][])
          n407 = local read "points in ellipse"() -> (w511:dbl)
          n408 = Build Array(w542, w541) -> (→"X-Y Graph 3":T1)
          n409 = local read "points in ellipse"() -> (w523:dbl)
          n410 = Array Size(array=w510) -> (size(s)=w515:i32)
          n411 = Array Size(array=w518) -> (size(s)=w519:i32)
          n412 = Decrement(x=w515) -> (x-1=w514:i32)
          n413 = Decrement(x=w519) -> (x-1=w520:i32)
          n414 = To Double Precision Float(number=w514) -> (double precision float=w513:dbl)
          n415 = To Double Precision Float(number=w520) -> (double precision float=w521:dbl)
          n416 = Divide(x=w513, y=w511) -> (x/y=w512:dbl)
          n417 = Divide(x=w521, y=w523) -> (x/y=w522:dbl)
          n418 = for {
            N: w511 -> [_]
            tunnel: w510 -> [w556]
            tunnel: w512 -> [w555]
            tunnel: [w554] -> w516 mode=indexing
            i -> [w552]
            n419 = Multiply(x=w555, y=w552) -> (x*y=w553:dbl)
            n420 = Interpolate 1D Array(1:w553, 2:w556) -> (0:w554:dbl)
          }
          n421 = for {
            N: w523 -> [_]
            tunnel: w518 -> [w561]
            tunnel: w522 -> [w560]
            tunnel: [w559] -> w517 mode=indexing
            i -> [w557]
            n422 = Multiply(x=w560, y=w557) -> (x*y=w558:dbl)
            n423 = Interpolate 1D Array(1:w558, 2:w561) -> (0:w559:dbl)
          }
          n424 = local write "Y-WaveArray"(w516) -> ()
          n425 = local write "X-WaveArray"(w517) -> ()
        }
      }
    }
  }
